vi "ADSR.vi"() -> ()   [LabVIEW 2014]
uses:
  State.ctl
  <vilib>/myRIO/Instrument Drivers/Onboard IO/AudioOut Block/typedefs/AudioOut Block Reference.ctl
  <vilib>/myRIO/Common/Instrument Driver Framework/Utilities/typedefs/myRIO Generic Hardware Reference.ctl
  <vilib>/myRIO/Common/Instrument Driver Framework/Utilities/typedefs/Hardware Version Enum.ctl
  <vilib>/myRIO/Common/Instrument Driver Framework/Utilities/typedefs/myRIO v1.0 Reference.ctl
  <vilib>/myRIO/Common/Instrument Driver Framework/Utilities/typedefs/Generic FPGA Reference.ctl
  <vilib>/myRIO/Common/Instrument Driver Framework/myRIO v1.0/AudioOut Block/typedefs/AudioOut Block Channels List.ctl
  <vilib>/myRIO/Common/Instrument Driver Framework/myRIO v1.0/AudioOut Block/typedefs/AudioOut Block Channels Enum.ctl
  <vilib>/myRIO/Common/Instrument Driver Framework/Utilities/typedefs/Analog Scaling Constants.ctl
  <vilib>/userdefined/High Color/nirio_resource_hc.ctl
  <vilib>/myRIO/Common/Instrument Driver Framework/Utilities/vis/Is FPGA Ref Available.vi
  <vilib>/myRIO/Common/Instrument Driver Framework/myRIO v1.0/AudioOut Block/vis/myRIO v1.1 Open Throughput AudioOut (N Samples).vi
  <vilib>/myRIO/Instrument Drivers/Onboard IO/AudioOut Block/vis/Write.vi
  <vilib>/myRIO/Common/Instrument Driver Framework/Utilities/vis/Validate Channels.vi
  <vilib>/Utility/VariantDataType/GetNumericInfo.vi
  <vilib>/Utility/error.llb/Error Cluster From Error Code.vi
  <vilib>/myRIO/Common/Instrument Driver Framework/myRIO v1.0/myRIO v1.1 Open Throughput.vi
  <vilib>/myRIO/Common/Instrument Driver Framework/myRIO v1.0/AudioOut Block/vis/myRIO v1.0 Get Scaling Constants AudioOut Block.vi
  <vilib>/myRIO/Common/Instrument Driver Framework/myRIO v1.0/AudioOut Block/vis/myRIO v1.0 Reserve AudioOut Block.vi
  <vilib>/myRIO/Common/Instrument Driver Framework/myRIO v1.0/Resource Manager/vis/myRIO v1.0 Open Writing DMA.vi
  <vilib>/myRIO/Common/Instrument Driver Framework/myRIO v1.0/myRIO v1.0 Close.vi
  <vilib>/myRIO/Common/Instrument Driver Framework/myRIO v1.0/AudioOut Block/vis/myRIO v1.0 AudioOut Block Write.vi
  <vilib>/myRIO/Express VI/Onboard IO/AudioOut/AudioOut Express VI.xnode
  <vilib>/myRIO/Instrument Drivers/Onboard IO/AudioOut Block/vis/myRIO AudioOut N Samples Open.xnode
  <vilib>/measure/NI_MABase.lvlib
  <vilib>/myRIO/Instrument Drivers/Onboard IO/AudioOut Block/AudioOut Block.lvlib
panel:
  out "End":bool
  out "End of Idle":i32=1002
  out "error out":errorcluster
  out "Gain Graph":dbl(graph)
  out "Gain":dbl
  out "Cicle Time (us)":u32(graph)=999
  in  "Pitch Frequency":dbl=2200.0 format="%#_13g"
  out "End Sustain":i32=2849
  out "Actual State":T1=enum."Release"
  in  "sampling info":cluster{"Fs":dbl, "#s":dbl}={"Fs"=10000.0, "#s"=1000.0} {"Fs" format="%.2p"}
  out "Waveform Chart":dbl[](graph)
  in  "Max. Amplitude (V)":dbl(slide)=0.7993311036789298 scale=0.0..1.0
  in  "Release (ms)":u32=500
  in  "Sustain (%)":dbl=60.0
  in  "Decay (ms)":u32=300
  in  "Attack (ms)":u32=1000
  in  "stop":bool
  in  "Activate":bool
  # "Envelope Filter"
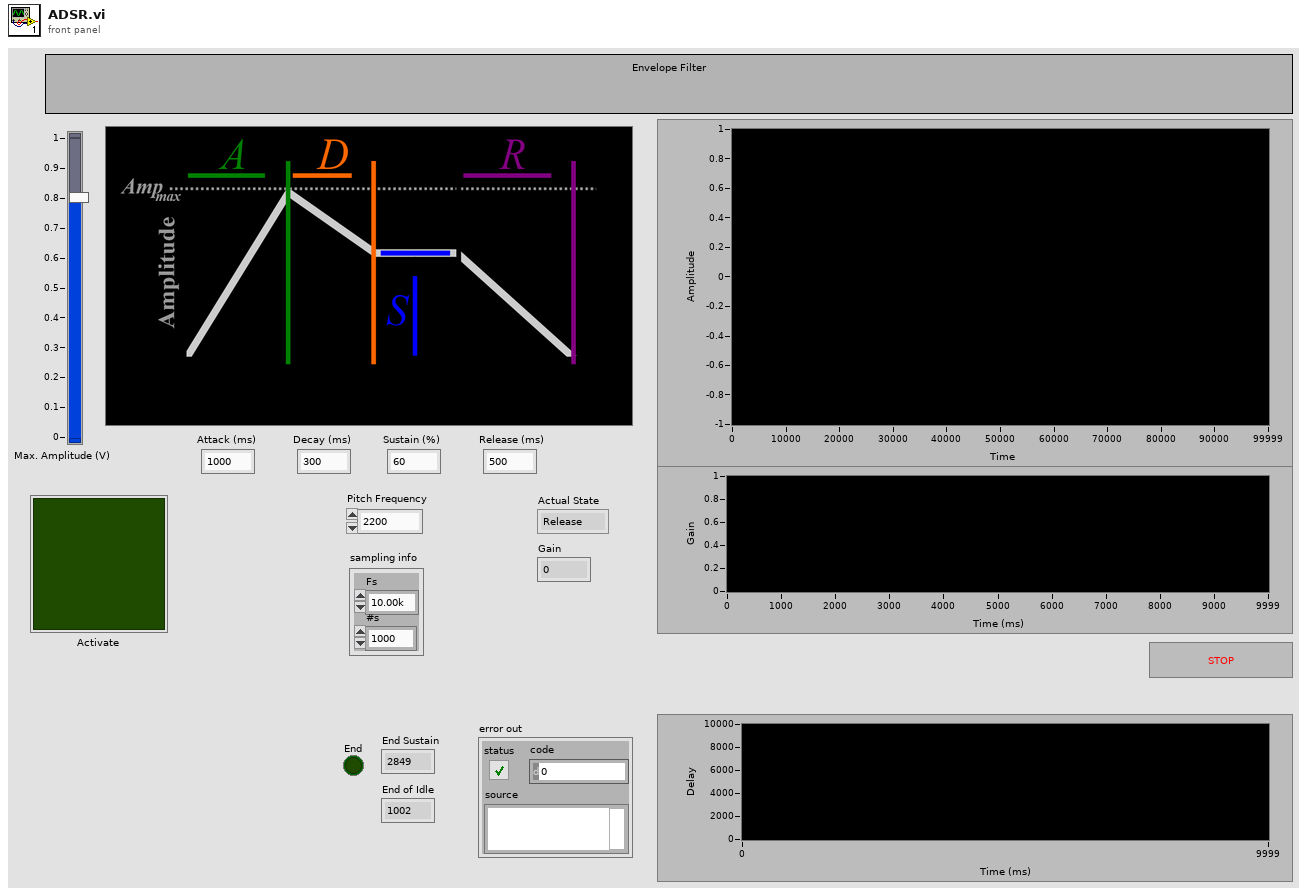
[diagram p1: front panel]
types:
  T1 = typedef "State.ctl" = enum16{"Idle", "Attack", "Decay", "Sustain", "Release"}
  T2 = typedef "AudioOut Block.lvlib/AudioOut Block Reference.ctl" = cluster{"myRIO Reference":T3, "AudioOut (N Samples) Channels List":T7, "AudioOut (N Samples) Scaling Constants List":T9[]}
  T3 = typedef "myRIO Generic Hardware Reference.ctl" = cluster{"myRIO Model":T4, "myRIO Hardware Reference":T5}
  T4 = typedef "Hardware Version Enum.ctl" = enum16{"Unknown", "myRIO-1900", "myRIO-1950"}
  T5 = typedef "myRIO v1.0 Reference.ctl" = cluster{"Generic FPGA Reference":T6, "Allow multiple opens":bool}
  T6 = typedef "Generic FPGA Reference.ctl" = refnum<k20>
  T7 = typedef "AudioOut Block Channels List.ctl" = T8[]
  T8 = typedef "AudioOut Block Channels Enum.ctl" = enum16{"Not Connected", "AudioOut/Left (N Samples)", "AudioOut/Right (N Samples)"}
  T9 = typedef "Analog Scaling Constants.ctl" = cluster{"LSB Weight (Volts)":dbl, "Offset (Volts)":dbl, "Signed?":bool}
  T10 = typedef "nirio_resource_hc.ctl" = tag
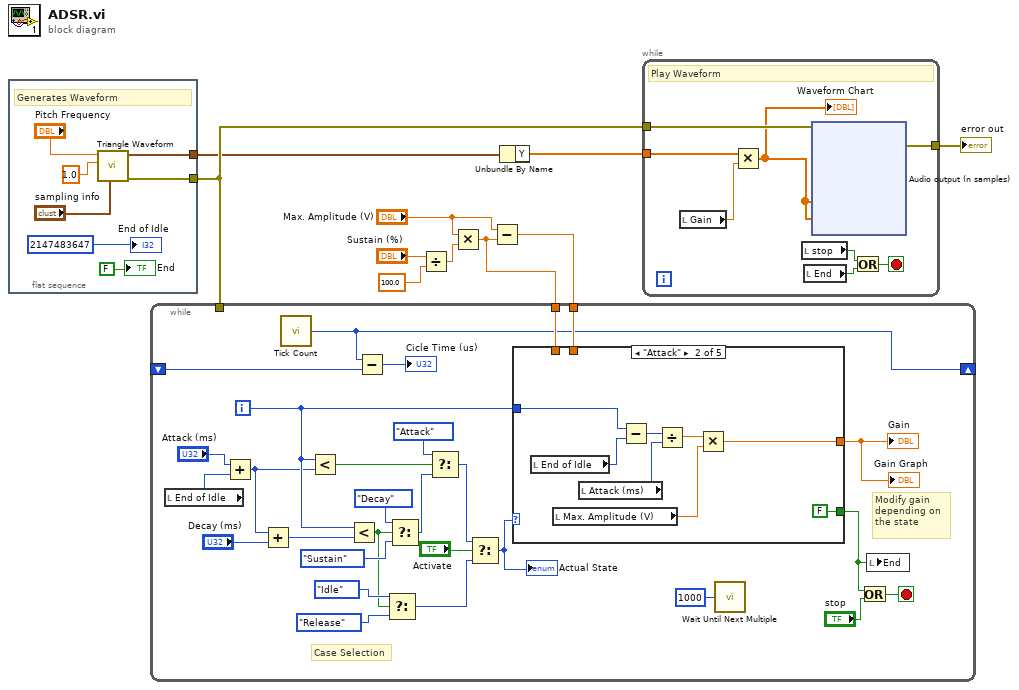
[diagram p0: block diagram]
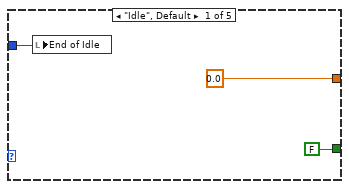
[diagram p2: hidden frame]
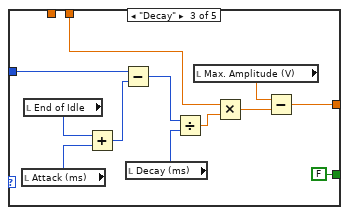
[diagram p3: hidden frame]
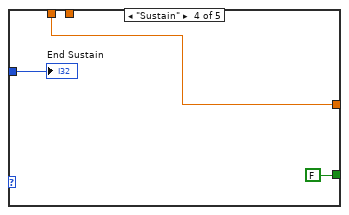
[diagram p4: hidden frame]
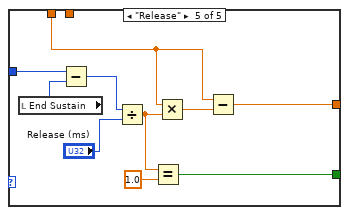
[diagram p5: hidden frame]
diagram:
  n1 = flat-sequence {
    tunnel: [w12] -> w1
    tunnel: [w13] -> w3
    frame #0 {
      # "Generates Waveform"
      n2 = call <vilib>:"Triangle Waveform.vi"("sampling info"="sampling info", "amplitude"=1.0, "frequency"="Pitch Frequency") -> ("error out"=w13:errorcluster, "signal out"=w12:waveform(dbl))  [unwired: 7 in]
      "End of Idle" <- 2147483647 ("End Sustain")
      "End" <- FALSE ("End")
    }
  }
  n3 = Divide(x="Sustain (%)", y=100.0) -> (x/y=w8:dbl)
  n4 = Multiply(x="Max. Amplitude (V)", y=w8) -> (x*y=w5:dbl)
  n5 = Subtract(x="Max. Amplitude (V)", y=w5) -> (x-y=w6:dbl)
  n6 = while {
    tunnel: w6 -> [w31]
    tunnel: w5 -> [w30]
    shift-right: [w27] -> _
    shift-left: _ -> [w26]
    tunnel: w3 -> [_]
    i -> [w39]
    stop <- w29 stop-if-true
    # "Modify gain\ndepending on\nthe state"
    # "Case Selection"
    n7 = local read "End of Idle"() -> (w19:i32)
    n8 = Add(x="Attack (ms)", y=w19) -> (x+y=w21:u32)
    n9 = Add(x=w21, y="Decay (ms)") -> (x+y=w20:u32)
    n10 = call "Tick Count"() -> ("Tick Count(uSec)"=w27:u32)
    n11 = Less?(x=w39, y=w21) -> (x < y?=w45:bool)
    n12 = Less?(x=w39, y=w20) -> (x < y?=w32:bool)
    n13 = Subtract(x=w27, y=w26) -> (x-y=→"Cicle Time (us)":u32)
    n14 = Select(t=State."Idle", s=w32, f=State."Release") -> (s? t:f=w35:T1)
    n15 = Select(t=State."Decay", s=w32, f=State."Sustain") -> (s? t:f=w41:T1)
    n16 = Select(t=State."Attack", s=w45, f=w41) -> (s? t:f=w43:T1)
    n17 = Select(t=w43, s="Activate", f=w35) -> (s? t:f=w37:T1)
    "Actual State" <- w37
    n18 = case shown="\"Attack\"" w37 {
      tunnel: w39 -> [w47 w52 w64 w70 w79]
      tunnel: w31 -> [_ _ w66 _ _]
      tunnel: w30 -> [_ _ _ w71 w77]
      tunnel: [FALSE ("End") FALSE ("End") FALSE ("End") FALSE ("End") w73] -> w18
      tunnel: [0.0 ("AudioOut/Left") w53 w61 w71 w72] -> w24
      frame "Idle", Default {
        n19 = local write "End of Idle"(w47) -> ()
      }
      frame "Attack" {
        n20 = local read "End of Idle"() -> (w51:i32)
        n21 = local read "Max. Amplitude (V)"() -> (w54:dbl)
        n22 = local read "Attack (ms)"() -> (w55:u32)
        n23 = Subtract(x=w52, y=w51) -> (x-y=w50:i32)
        n24 = Divide(x=w50, y=w55) -> (x/y=w56:dbl)
        n25 = Multiply(x=w56, y=w54) -> (x*y=w53:dbl)
      }
      frame "Decay" {
        n26 = local read "Attack (ms)"() -> (w59:u32)
        n27 = local read "End of Idle"() -> (w58:i32)
        n28 = Add(x=w58, y=w59) -> (x+y=w60:u32)
        n29 = Subtract(x=w64, y=w60) -> (x-y=w62:u32)
        n30 = local read "Decay (ms)"() -> (w63:u32)
        n31 = Divide(x=w62, y=w63) -> (x/y=w65:dbl)
        n32 = local read "Max. Amplitude (V)"() -> (w67:dbl)
        n33 = Multiply(x=w66, y=w65) -> (x*y=w68:dbl)
        n34 = Subtract(x=w67, y=w68) -> (x-y=w61:dbl)
      }
      frame "Sustain" {
        "End Sustain" <- w70
      }
      frame "Release" {
        n35 = local read "End Sustain"() -> (w76:i32)
        n36 = Subtract(x=w79, y=w76) -> (x-y=w80:i32)
        n37 = Divide(x=w80, y="Release (ms)") -> (x/y=w75:dbl)
        n38 = Equal?(x=w75, y=1.0) -> (x = y?=w73:bool)
        n39 = Multiply(x=w77, y=w75) -> (x*y=w81:dbl)
        n40 = Subtract(x=w77, y=w81) -> (x-y=w72:dbl)
      }
    }
    "Gain Graph" <- w24
    "Gain" <- w24
    n41 = call "Wait Until Next Multiple"("Count(uSec)"=u32 1000) -> ()  [unwired: 1 out]
    n42 = Or(x=w18, y="stop") -> (x .or. y?=w29:bool)
    n43 = local write "End"(w18) -> ()
  }
  n44 = Unbundle By Name(w1) -> ("Y"=w4:dbl[])
  n45 = while {
    tunnel: w4 -> [w84]
    tunnel: w3 -> [w88]
    tunnel: [w89] -> w2
    stop <- w87 stop-if-true
    # "Play Waveform"
    n46 = local read "Gain"() -> (w83:dbl)
    n47 = Multiply(x=w84, y=w83) -> (x*y=w82:dbl[])
    "Waveform Chart" <- w82
    n48 = local read "stop"() -> (w86:bool)
    n49 = local read "End"() -> (w85:bool)
    n50 = xnode "Audio output (n samples)"("AudioOut/Left (N Samples)"=w82, "AudioOut/Right (N Samples)"=w82, "error in (no error)"=w88) -> ("error out"=w89:errorcluster)
    n51 = Or(x=w86, y=w85) -> (x .or. y?=w87:bool)
  }
  "error out" <- w2
